vi "Closed Loop Verification.vi"(8 "Allowable Error Factor":dbl=0.02 format="%#_13g", 10 "Actual":dbl, 11 "Target":dbl) -> (2 "At Target w/in Allowable Error?":bool)   [LabVIEW 2015]
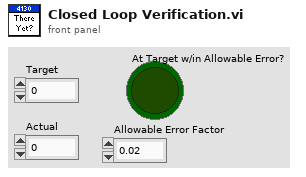
[diagram p1: front panel]
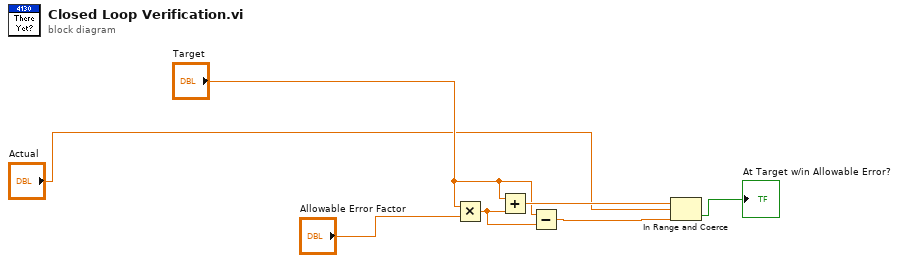
[diagram p0: block diagram]
diagram:
  n1 = Multiply(x="Target", y="Allowable Error Factor") -> (x*y=w5:dbl)
  n2 = Add(x="Target", y=w5) -> (x+y=w4:dbl)
  n3 = Subtract(x="Target", y=w5) -> (x-y=w6:dbl)
  n4 = In Range and Coerce(upper limit=w4, x="Actual", lower limit=w6) -> (In Range?=→"At Target w/in Allowable Error?":bool)  [unwired: 1 out]
